vi "Set_PRR.vi"(8 "error in (no error)":errorcluster, 10 "PRR":sgl, 11 "connection ID":refnum<k5>) -> (0 "error out":errorcluster, 2 "Checksum OK":bool, 3 "connection ID out":refnum<k5>)   [LabVIEW 2023, in "Laser_com_2022.lvlib"]
uses:
  Laser_com_2022.lvlib
panel:
  out "Data":string
  out "data in":string
  out "length":i32
  out "Data size":u32
  out "Execution code`":u16
  out "Answer":u16
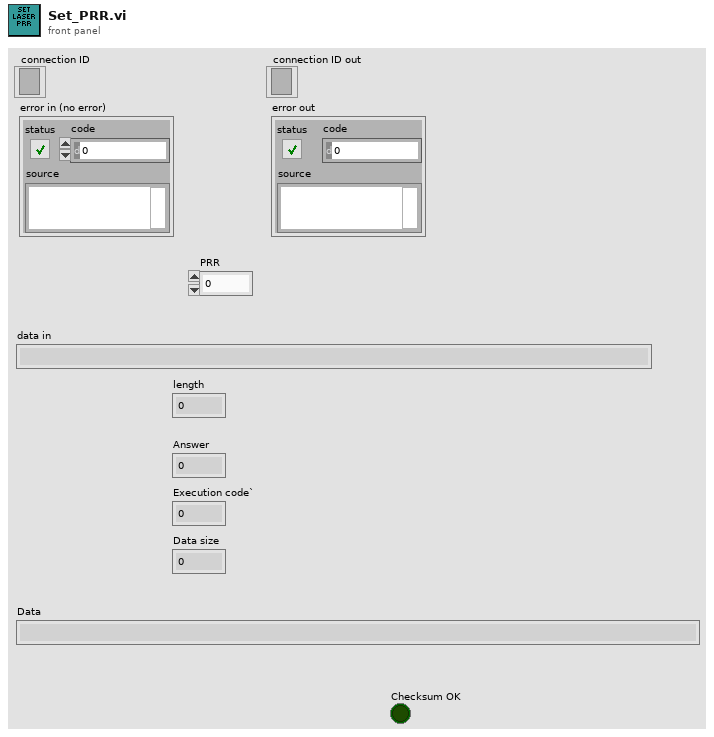
[diagram p1: front panel]
types:
  T1 = enum16{"big-endian, network order", "native, host order", "little-endian"}
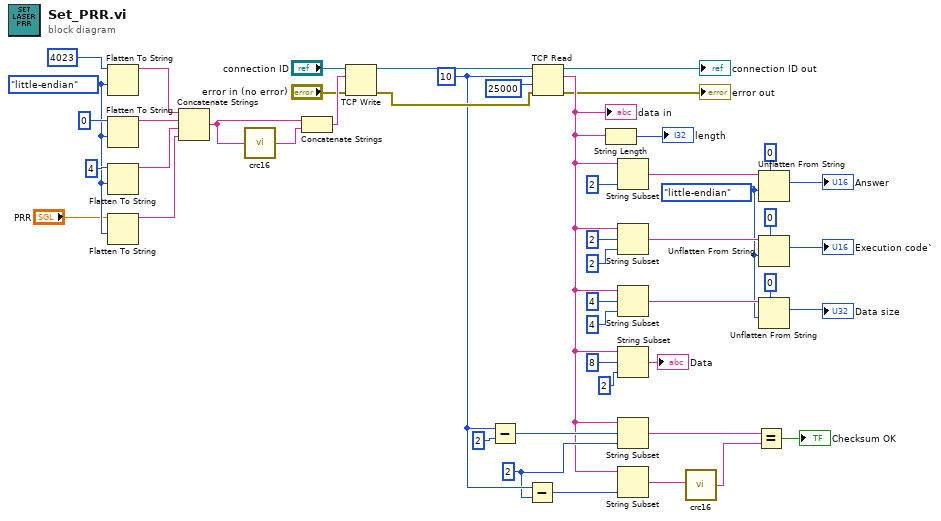
[diagram p0: block diagram]
diagram:
  w15 = T1."little-endian" ("byte order (0:big-endian, network order)")
  w3 = T1."little-endian" ("byte order (0:big-endian, network order)")
  w34 = 2 ("length (rest)")
  w35 = 10 ("bytes to read")
  n1 = Flatten To String(anything=u16 4023 ("Command"), byte order (0:big-endian, network order)=w3) -> (data string=w29:string)  [unwired: 2 in, 2 out]
  n2 = Flatten To String(anything=u16 0, byte order (0:big-endian, network order)=w3) -> (data string=w28:string)  [unwired: 2 in, 2 out]
  n3 = Flatten To String(anything=u32 4 ("Datasize"), byte order (0:big-endian, network order)=w3) -> (data string=w27:string)  [unwired: 2 in, 2 out]
  n4 = Flatten To String(anything="PRR", byte order (0:big-endian, network order)=w3) -> (data string=w2:string)  [unwired: 2 in, 2 out]
  n5 = Concatenate Strings(w29, w28, w27, w2) -> (w10:string)
  n6 = call "crc16.vi"("string"=w10) -> ("string 2"=w11:string)
  n7 = Concatenate Strings(w10, w11) -> (w43:string)
  n8 = TCP Write(connection ID="connection ID", data in=w43, error in (no error)="error in (no error)") -> (connection ID out=w48:refnum<k5>, error out=w46:errorcluster)  [unwired: 1 in, 1 out]
  n9 = Subtract(x=w35, y=2 ("offset (0)")) -> (x-y=w37:i32)
  n10 = Subtract(x=w35, y=w34) -> (x-y=w33:i32)
  n11 = TCP Read(connection ID=w48, bytes to read=w35, error in (no error)=w46, 9:25000 ("timeout ms (25000)")) -> (connection ID out=→"connection ID out":refnum<k5>, data out=w26:string, error out=→"error out":errorcluster)  [unwired: 1 in]
  "data in" <- w26
  n12 = String Length(string=w26) -> (length=→"length":i32)
  n13 = String Subset(string=w26, length (rest)=2 ("length (rest)")) -> (substring=w21:string)  [unwired: 1 in]
  n14 = String Subset(string=w26, offset (0)=2, length (rest)=2 ("length (rest)")) -> (substring=w19:string)
  n15 = String Subset(string=w26, offset (0)=4, length (rest)=4 ("length (rest)")) -> (substring=w16:string)
  n16 = String Subset(string=w26, offset (0)=8, length (rest)=2 ("length (rest)")) -> (substring=→"Data":string)
  n17 = String Subset(string=w26, offset (0)=w37, length (rest)=w34) -> (substring=w36:string)
  n18 = String Subset(string=w26, length (rest)=w33) -> (substring=w9:string)  [unwired: 1 in]
  n19 = call "crc16.vi"("string"=w9) -> ("string 2"=w6:string)
  n20 = Equal?(x=w36, y=w6) -> (x = y?=→"Checksum OK":bool)
  n21 = Unflatten From String(type=u16 0, binary string=w21, byte order (0:big-endian, network order)=w15) -> (value=→"Answer":u16)  [unwired: 2 in, 2 out]
  n22 = Unflatten From String(type=u16 0, binary string=w19, byte order (0:big-endian, network order)=w15) -> (value=→"Execution code`":u16)  [unwired: 2 in, 2 out]
  n23 = Unflatten From String(type=u32 0, binary string=w16, byte order (0:big-endian, network order)=w15) -> (value=→"Data size":u32)  [unwired: 2 in, 2 out]
